vi "Set_5G_Tracking_Area_Code.vi"(8 "error in (no error)":errorcluster, 10 "value":i64=1 min=0 max=65535, 11 "Base Station":T1) -> (0 "error out":errorcluster, 3 "Output String":string)   [LabVIEW 2021]
uses:
  Controls/Base_Station_Emulator.ctl
  Controls/TCP_FGV.ctl
panel:
  # "The possible values \nare from 0 to 65535. \n The default value is 1."
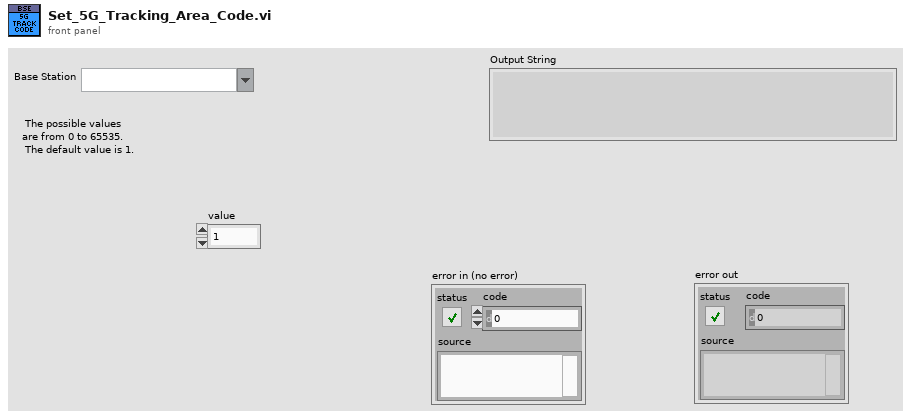
[diagram p1: front panel]
types:
  T1 = typedef "Base_Station_Emulator.ctl" = string
  T2 = typedef "TCP_FGV.ctl" = enum16{"Open", "Read", "Write", "Close"}
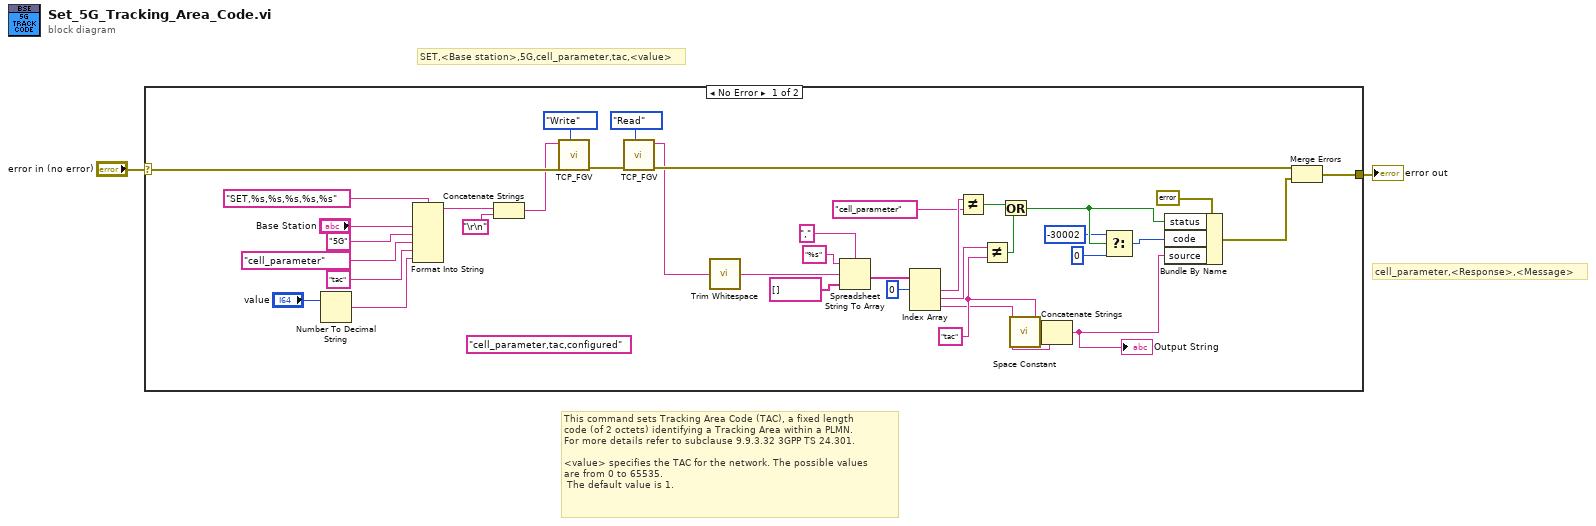
[diagram p0: block diagram]
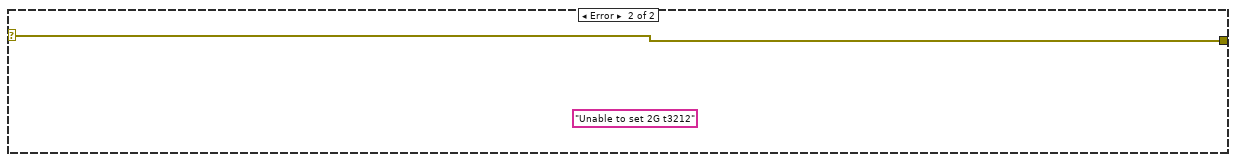
[diagram p2: hidden frame]
diagram:
  # "This command sets Tracking Area Code (TAC), a fixed length \ncode (of 2 octets) identifying a Tracking Area within a PLMN. \nFor more details refer to subclause 9.9.3.32 3GPP TS 24.301. \n\n<value> specifies the TAC for the network. The possible values \nare from 0 to 65535. \n The default value is 1."
  # "SET,<Base station>,5G,cell_parameter,tac,<value>"
  # "cell_parameter,<Response>,<Message>"
  n1 = case shown="No Error" "error in (no error)" {
    selector: "error in (no error)" -> [w37 w41]
    tunnel: [w15 w41] -> w1
    frame No Error {
      (unwired) "cell_parameter,tac,configured" ("format string")
      w13 = "tac"
      n2 = Number To Decimal String(number="value") -> (decimal integer string=w4:string)  [unwired: 1 in]
      n3 = Format Into String(format string="SET,%s,%s,%s,%s,%s", "Base Station", "5G", "cell_parameter", "tac", w4) -> (resulting string=w7:string)  [unwired: 2 in, 1 out]
      n4 = Concatenate Strings(w7, "\r\n") -> (w6:string)
      n5 = call "TCP_FGV.vi"("Command"=w6, "error in (no error)"=w37, "Operation"=TCP_FGV."Write") -> ("error out"=w16:errorcluster)  [unwired: 6 in, 1 out]
      n6 = call "TCP_FGV.vi"("error in (no error)"=w16, "Operation"=TCP_FGV."Read") -> ("Data Out"=w3:string, "error out"=w18:errorcluster)  [unwired: 7 in]
      n7 = call <vilib>:"Trim Whitespace.vi"("string"=w3) -> ("trimmed string"=w32:string)  [unwired: 1 in]
      n8 = Spreadsheet String To Array(delimiter (Tab)=",", format string="%s", spreadsheet string=w32, array type (2D Dbl)=string[] []) -> (array=w28:string[])
      n9 = Index Array(array=w28, index #1=0 ("index")) -> (element #1=w29:string, element #2=w19:string, element #3=w12:string)  [unwired: 2 in]
      n10 = Not Equal?(x=w29, y="cell_parameter" ("format string")) -> (x != y?=w30:bool)
      n11 = Not Equal?(x=w19, y=w13) -> (x != y?=w31:bool)
      n12 = Or(x=w30, y=w31) -> (x .or. y?=w33:bool)
      n13 = call <vilib>:"Space Constant.vi"() -> ("String"=w14:string)
      n14 = Concatenate Strings(w13, w14, w12) -> (w11:string)
      "Output String" <- w11
      n15 = Select(t=-30002 ("code"), s=w33, f=0 ("code")) -> (s? t:f=w34:i32)
      n16 = Bundle By Name(cluster=errorcluster {"status"=FALSE, "code"=0, "source"=""} ("error constant"), "status"=w33, "code"=w34, "source"=w11) -> (w17:errorcluster)
      n17 = Merge Errors(w18, w17) -> (w15:errorcluster)
    }
    frame Error {
      (unwired) "Unable to set 2G t3212" ("source")
    }
  }
  "error out" <- w1
